vi "Station_Port_Dialog_Serial.vi"(5 "Enable":bool=TRUE, 7 "Error in":errorcluster, 8 "Station ID in":i32 min=0, 9 "Baud rate in":i32(ring)=19200 items=["1200"=1200, "2400"=2400, "4800"=4800, "9600"=9600, "14400"=14400, "19200"=19200], 10 "COM port in":i32 min=0) -> (0 "Error out":errorcluster, 1 "Station ID out":i32, 2 "Baud rate out":i32, 3 "COM port out":i32, 4 "OK":bool, 6 "Help?":bool)   [LabVIEW 2012]
doc: "Displays a standard dialog box that prompts users to enter information, such as a user name and password.\n--------------------\n\nThis Express VI is configured as follows:\n\nMessage to Display to the User:There is a problem in communication with the Vantage Pro console. Check if the console is properly connected with your PC and that you selected the correct COM port number (you can find this number at 'device manager' (apparaatbeheer)).\n\nMoreover select the correct baud rate (19200).\n\nFinally, select the HiSPARC Station ID in (you can find your ID in the file 'Z:\\persistent\\config.ini').\nThe inputs are: \nNumber: COM Poort\nNumber: Baud rate\nNumber: Station ID"
panel:
  in  "Baud rate":i32(ring)=19200 items=["1200"=1200, "2400"=2400, "4800"=4800, "9600"=9600, "14400"=14400, "19200"=19200]
  in  "Station ID":i32 min=0
  in  "COM port":i32 caption="COM Poort" min=0 step=1
  in  "OK":bool
  in  "Stop?":bool
  in  "Help?":bool
  out "String":string="Please select to connect:\n\n- COM port number\n  - Launch the Windows 'Device Manager' (Apparatenbeheer)\n  - Open 'COM & LPT'\n  - Windows assigned a 'COM number' for your serial connection\n\n- Baud rate\n  - Speed at which your weather station communicates with your computer\n  - Default: 19200\n\n- Station ID\n  - Identifier for your station distributed together with your certificate\n    (required during software installation)\n  - Usually the same ID as your cosmic ray detector\n  - The ID of your cosmic ray station is stored in: \\persistent\\config.ini"
  in  "OK1":bool
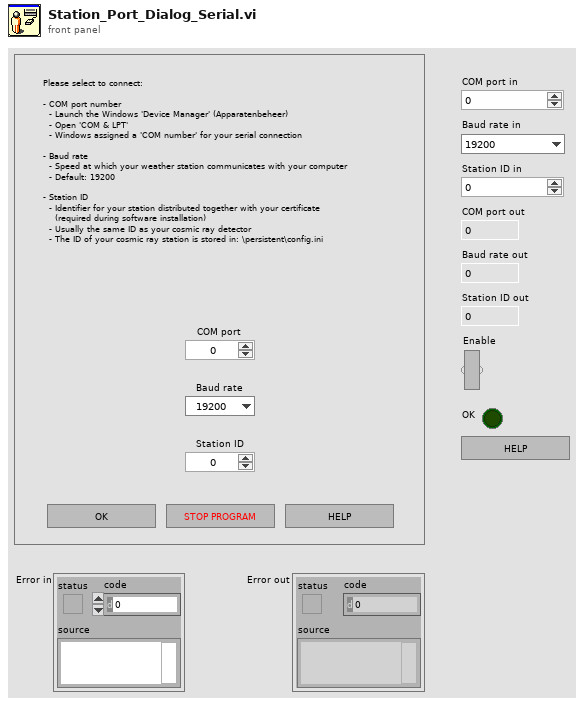
[diagram p1: front panel]
types:
  T1 = cluster{"Input Name":string, "Input Data Type":i32}[]
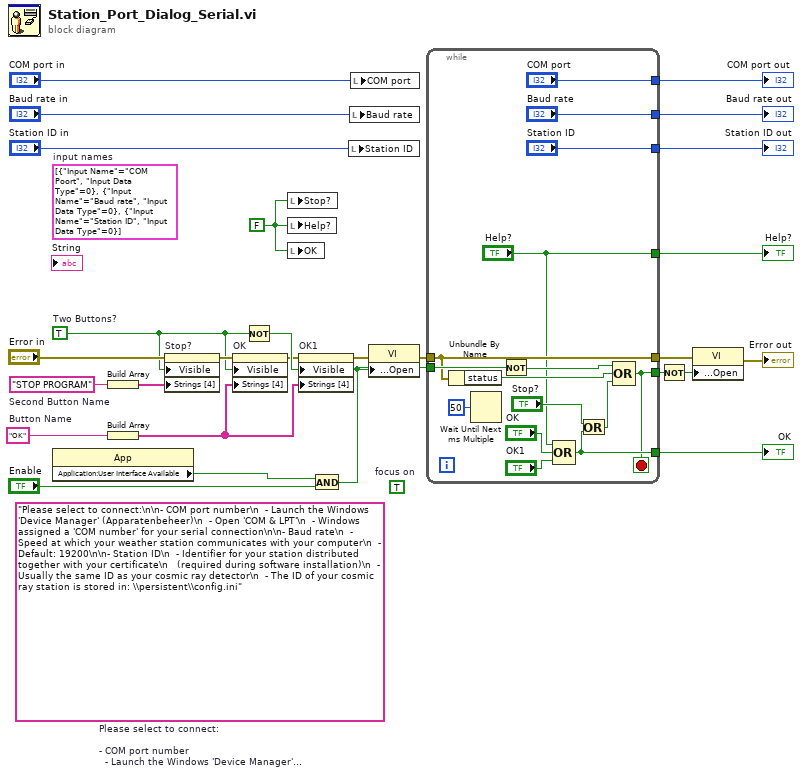
[diagram p0: block diagram]
diagram:
  w1 = FALSE ("Help?")
  (unwired) "Please select to connect:\n\n- COM port number\n  - Launch the Windows 'Device Manager' (Apparatenbeheer)\n  - Open 'COM & LPT'\n  - Windows assigned a 'COM number' for your serial connection\n\n- Baud rate\n  - Speed at which your weather station communicates with your computer\n  - Default: 19200\n\n- Station ID\n  - Identifier for your station distributed together with your certificate\n   (required during software installation)\n  - Usually the same ID as your cosmic ray detector\n  - The ID of your cosmic ray station is stored in: \\persistent\\config.ini"  # Please select to connect:  - COM port number   - Launch the Windows 'Device Manager' (Apparatenbeheer)   - Open 'COM & LPT'   - Windows assigned a 'COM number' for your serial connection  - Baud rate   - Speed at which your weather station communicates with your computer   - Default: 19200  - Station ID   - Identifier for your station distributed together with your certificate    (required during software installation)   - Usually the same ID as your cosmic ray detector   - The ID of your cosmic ray station is stored in: \persistent\config.ini
  (unwired) TRUE  # focus on
  (unwired) T1 [{"Input Name"="COM Poort", "Input Data Type"=0}, {"Input Name"="Baud rate", "Input Data Type"=0}, {"Input Name"="Station ID", "Input Data Type"=0}]  # input names
  w23 = "STOP PROGRAM"  # Second Button Name
  w22 = "OK"  # Button Name
  w5 = TRUE  # Two Buttons?
  n1 = property class="App"() -> ("Application:User Interface Available"=w10:bool)  [unwired: 2 in, 2 out]
  n2 = Build Array(w23) -> (w7:string[])
  n3 = Build Array(w22) -> (w3:string[])
  n4 = property on="Stop?" class="Bool (strict)"(error in="Error in", "Visible"=w5, "Strings [4]"=w7) -> (error out=w6:errorcluster)  [unwired: 1 in, 1 out]
  n5 = property on="OK" class="Bool (strict)"(error in=w6, "Visible"=w5, "Strings [4]"=w3) -> (error out=w4:errorcluster)  [unwired: 1 in, 1 out]
  n6 = Not(x=w5) -> (.not. x?=w26:bool)
  n7 = local write "Stop?"(w1) -> ()
  n8 = local write "Help?"(w1) -> ()
  n9 = local write "OK"(w1) -> ()
  n10 = property on="OK1" class="Bool"(error in=w4, "Visible"=w26, "Strings [4]"=w3) -> (error out=w21:errorcluster)  [unwired: 1 in, 1 out]
  n11 = And(x=w10, y="Enable") -> (x .and. y?=w17:bool)
  n12 = local write "Station ID"("Station ID in") -> ()
  n13 = local write "Baud rate"("Baud rate in") -> ()
  n14 = local write "COM port"("COM port in") -> ()
  n15 = property class="VI"(error in=w21, "Front Panel Window:Open"=w17) -> (error out=w20:errorcluster)  [unwired: 1 in, 1 out]
  n16 = while "Main While Loop" {
    tunnel: [w41] -> w27
    tunnel: w17 -> [w40]
    tunnel: [w38] -> w24
    tunnel: w20 -> [w37]
    tunnel: [w37] -> w19
    tunnel: ["COM port"] -> w16
    tunnel: ["Baud rate"] -> w15
    tunnel: ["Station ID"] -> w14
    tunnel: ["Help?"] -> w2
    stop <- w38 stop-if-true
    n17 = Unbundle By Name(w37) -> ("status"=w35:bool)
    n18 = Wait Until Next ms Multiple(millisecond multiple=u32 50) -> ()  [unwired: 1 out]
    n19 = Not(x=w40) -> (.not. x?=w39:bool)
    n20 = Compound Arithmetic op=OR("Help?", "OK", "OK1") -> (w41:bool)
    n21 = Or(x="Stop?", y=w41) -> (x .or. y?=w36:bool)
    n22 = Compound Arithmetic op=OR(w39, w35, w36) -> (w38:bool)
  }
  "OK" <- w27
  "COM port out" <- w16
  "Baud rate out" <- w15
  "Station ID out" <- w14
  "Help?" <- w2
  n23 = Not(x=w24) -> (.not. x?=w25:bool)
  n24 = property class="VI"(error in=w19, "Front Panel Window:Open"=w25) -> (error out=→"Error out":errorcluster)  [unwired: 1 in, 1 out]
